vi "run _time_fgv .vi"(2 "error in (no error)":errorcluster, 3 "mode":enum16{"read", "write"}(ring), 4 "Value  in":T1) -> (0 "error out":errorcluster, 1 "Value out":T1)   [LabVIEW 2019]
uses:
  profile value.ctl
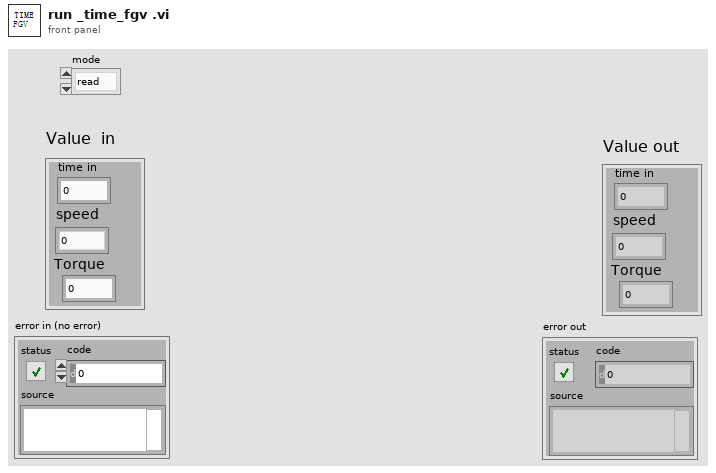
[diagram p1: front panel]
types:
  T1 = typedef "profile value.ctl" = cluster{"time in":i32, "speed":dbl, "Torque":dbl}
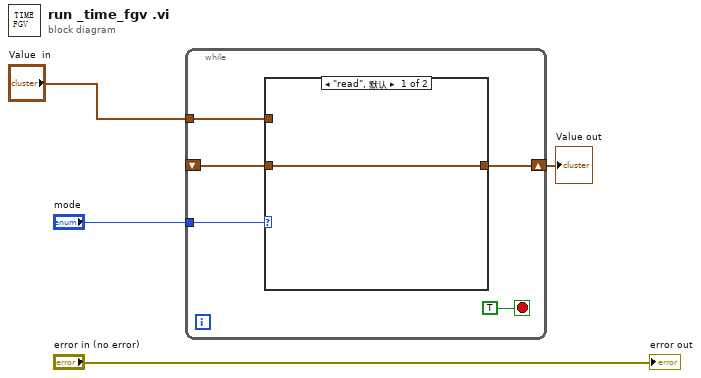
[diagram p0: block diagram]
diagram:
  n1 = while {
    tunnel: "mode" -> [w9]
    tunnel: "Value  in" -> [w8]
    shift-right: [w7] -> w1
    shift-left: _ -> [w6]
    stop <- TRUE stop-if-true
    n2 = case shown="\"read\", 默认" w9 {
      tunnel: [w10 w11] -> w7
      tunnel: w8 -> [_ w11]
      tunnel: w6 -> [w10 _]
      frame "read", Default {
      }
      frame "write" {
      }
    }
  }
  "Value out" <- w1
  "error out" <- "error in (no error)"
